vi "TapeMonitor_new.vi"() -> ()   [LabVIEW 2013]
uses:
  shared programs/GUI_Template/GUI_master/tcp_new_data_event.ctl
  shared programs/GUI_Template/GUI_master/tcp new data cluster.ctl
  <vilib>/vision/Image Controls.llb/IMAQ Image.ctl
  <vilib>/vision/NI_Vision_Development_Module.lvlib
  <vilib>/Analysis/NI_AALBase.lvlib
panel:
  out "x-y":dbl=0.8
  out "sqrt(x)":dbl=nan
  out "fitness":dbl=nan
  out "area symmetry":dbl=nan
  out "standard deviation":dbl=-0.0 format="%0.2f"
  out "Array":dbl[](array[numeric])
  out "symmetry":dbl=nan
  out "Number of Particles":i32
  out "X":dbl[](array[numeric])
  out "Y":dbl[](array[numeric])
  in  "Font, Size & Style":T1={"Desired Font (Application)"=enum."Application Font", "[User-specified Font]"={"Font Name"="", "Size"=12, "Strikeout?"=FALSE, "Italic?"=FALSE, "Underline?"=FALSE, "Outline?"=FALSE, "Shadow?"=FALSE, "Bold?"=FALSE, "Rotation Angle"=0.0}, "Horizontal Alignment"=0, "Vertical Alignment"=0} {"Vertical Alignment" items=["Bottom", "Top", "Baseline"]; "Horizontal Alignment" items=["Left", "Center", "Right"]; "[User-specified Font]"."Rotation Angle" format="%.2f"}
  in  "Selection Values":T3(array[cluster])=[{"Measurement Parameter"=35, "Range Lower Value"=0.0, "Range Upper Value"=500.0, "Range"=TRUE, "Measurement Type"=FALSE}] {"Measurement Parameter" items=["Center of Mass X", "Center of Mass Y", "First Pixel X", "First Pixel Y", "Bounding Rect Left", "Bounding Rect Top", "Bounding Rect Right", "Bounding Rect Bottom", "Max Feret Diameter Start X", "Max Feret Diameter Start Y", "Max Feret Diameter End X", "Max Feret Diameter End Y", "Max Horiz. Segment Length Left", "Max Horiz. Segment Length Right", "Max Horiz. Segment Length Row", "-", "Bounding Rect Width", "Bounding Rect Height", "Bounding Rect Diagonal", "Perimeter", "Convex Hull Perimeter", "Holes' Perimeter", "Max Feret Diameter", "Equivalent Ellipse Major Axis", "Equivalent Ellipse Minor Axis", "Equivalent Ellipse Minor Axis (Feret)", "Equivalent Rect Long Side", "Equivalent Rect Short Side", "Equivalent Rect Diagonal", "Equivalent Rect Short Side (Feret)", "Average Horiz. Segment Length", "Average Vert. Segment Length", "Hydraulic Radius", "Waddel Disk Diameter", "-", "Area", "Holes' Area", "Particle & Holes' Area", "Convex Hull Area", "Image Area", "-", "Number of Holes", "Number of Horiz. Segments", "Number of Vert. Segments", "-", "Orientation", "Max Feret Diameter Orientation", "-", "% Area/Image Area", "% Area/(Particle & Holes' Area)", "Ratio of Equivalent Ellipse Axes", "Ratio of Equivalent Rect Sides", "-", "Elongation Factor", "Compactness Factor", "Heywood Circularity Factor", "Type Factor", "-", "Sum X", "Sum Y", "Sum XX", "Sum XY", "Sum YY", "Sum XXX", "Sum XXY", "Sum XYY", "Sum YYY", "-", "Moment of Inertia XX", "Moment of Inertia XY", "Moment of Inertia YY", "Moment of Inertia XXX", "Moment of Inertia XXY", "Moment of Inertia XYY", "Moment of Inertia YYY", "Norm. Moment of Inertia XX", "Norm. Moment of Inertia XY", "Norm. Moment of Inertia YY", "Norm. Moment of Inertia XXX", "Norm. Moment of Inertia XXY", "Norm. Moment of Inertia XYY", "Norm. Moment of Inertia YYY", "Hu Moment 1", "Hu Moment 2", "Hu Moment 3", "Hu Moment 4", "Hu Moment 5", "Hu Moment 6", "Hu Moment 7"]}
  in  "Keep/Replace Value (Replace) 2":bool=TRUE
  out "image2":T4(plugin-control) caption="Mode1"
  in  "Size & Order # 2":T5={"X Size"=3, "Y Size"=3, "Order #"=8}
  in  "Range 2":cluster{"Lower value":sgl, "Upper value":sgl}={"Lower value"=140.0, "Upper value"=255.0} {"Upper value" format="%.2f"; "Lower value" format="%.2f"}
  in  "gain::1":dbl caption="gain" min=0.0 max=12.0 format="%_4p"
  out "image::1":T4(plugin-control) caption="Mode1"
  in  "exposure::1":dbl=0.01 caption="Exposure" min=0.0001 max=1.0 format="%_4p"
  in  "insert tag":bool=TRUE
  in  "stop":bool
  in  "trigger::1":bool caption="Trigger"
  in  "GUIdevice 1":string="StagingTapeMonitorCam"
  out "tcp data event":T6
  out "error IO 2":errorcluster
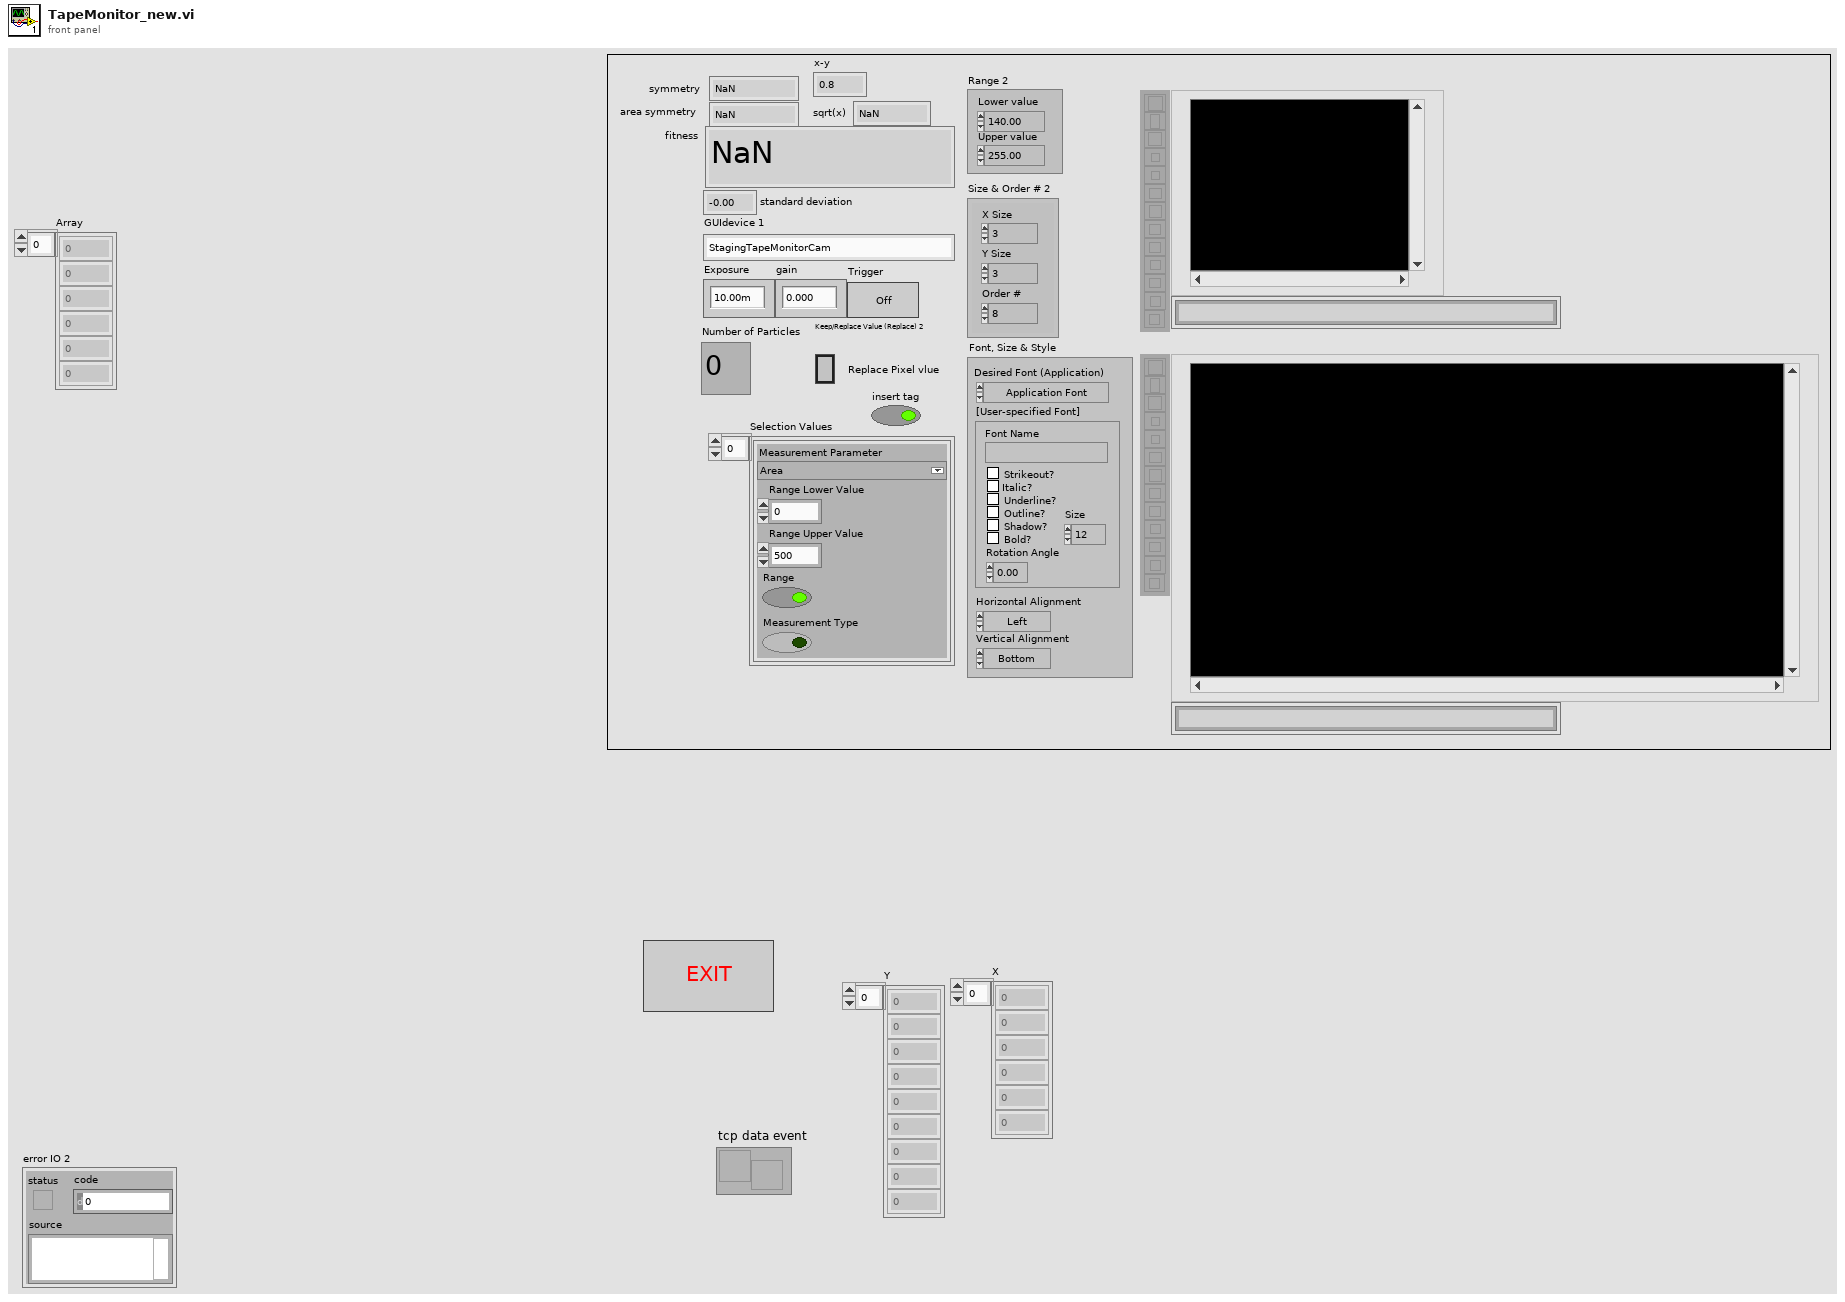
[diagram p1: front panel]
types:
  T1 = cluster{"Desired Font (Application)":enum16{"User-specified Font", "Application Font", "System Font", "Dialog Font"}, "[User-specified Font]":cluster{"Font Name":string, "Size":i16, "Strikeout?":bool, "Italic?":bool, "Underline?":bool, "Outline?":bool, "Shadow?":bool, "Bold?":bool, "Rotation Angle":dbl}, "Horizontal Alignment":i16, "Vertical Alignment":i16}
  T2 = typedef "Particle Parameters" = i32
  T3 = cluster{"Measurement Parameter":T2, "Range Lower Value":dbl, "Range Upper Value":dbl, "Range":bool, "Measurement Type":bool}[]
  T4 = typedef "IMAQ Image.ctl" = refnum<image>
  T5 = cluster{"X Size":i32, "Y Size":i32, "Order #":i32}
  T6 = typedef "tcp_new_data_event.ctl" = refnum<user-event>
  T7 = typedef "Image Type" = u32
  T8 = typedef "tcp new data cluster.ctl" = cluster{"EventEnum":enum16{"new data", "connection status update"}, "Device name":string}
  T9 = cluster{"Particle Measurements (Pixels)[0]":dbl, "Particle Measurements (Pixels)[1]":dbl, "Particle Measurements (Pixels)[2]":dbl, "Particle Measurements (Pixels)[3]":dbl}
  T10 = cluster{"Particle Measurements (Pixels)[0]":dbl, "Particle Measurements (Pixels)[1]":dbl}
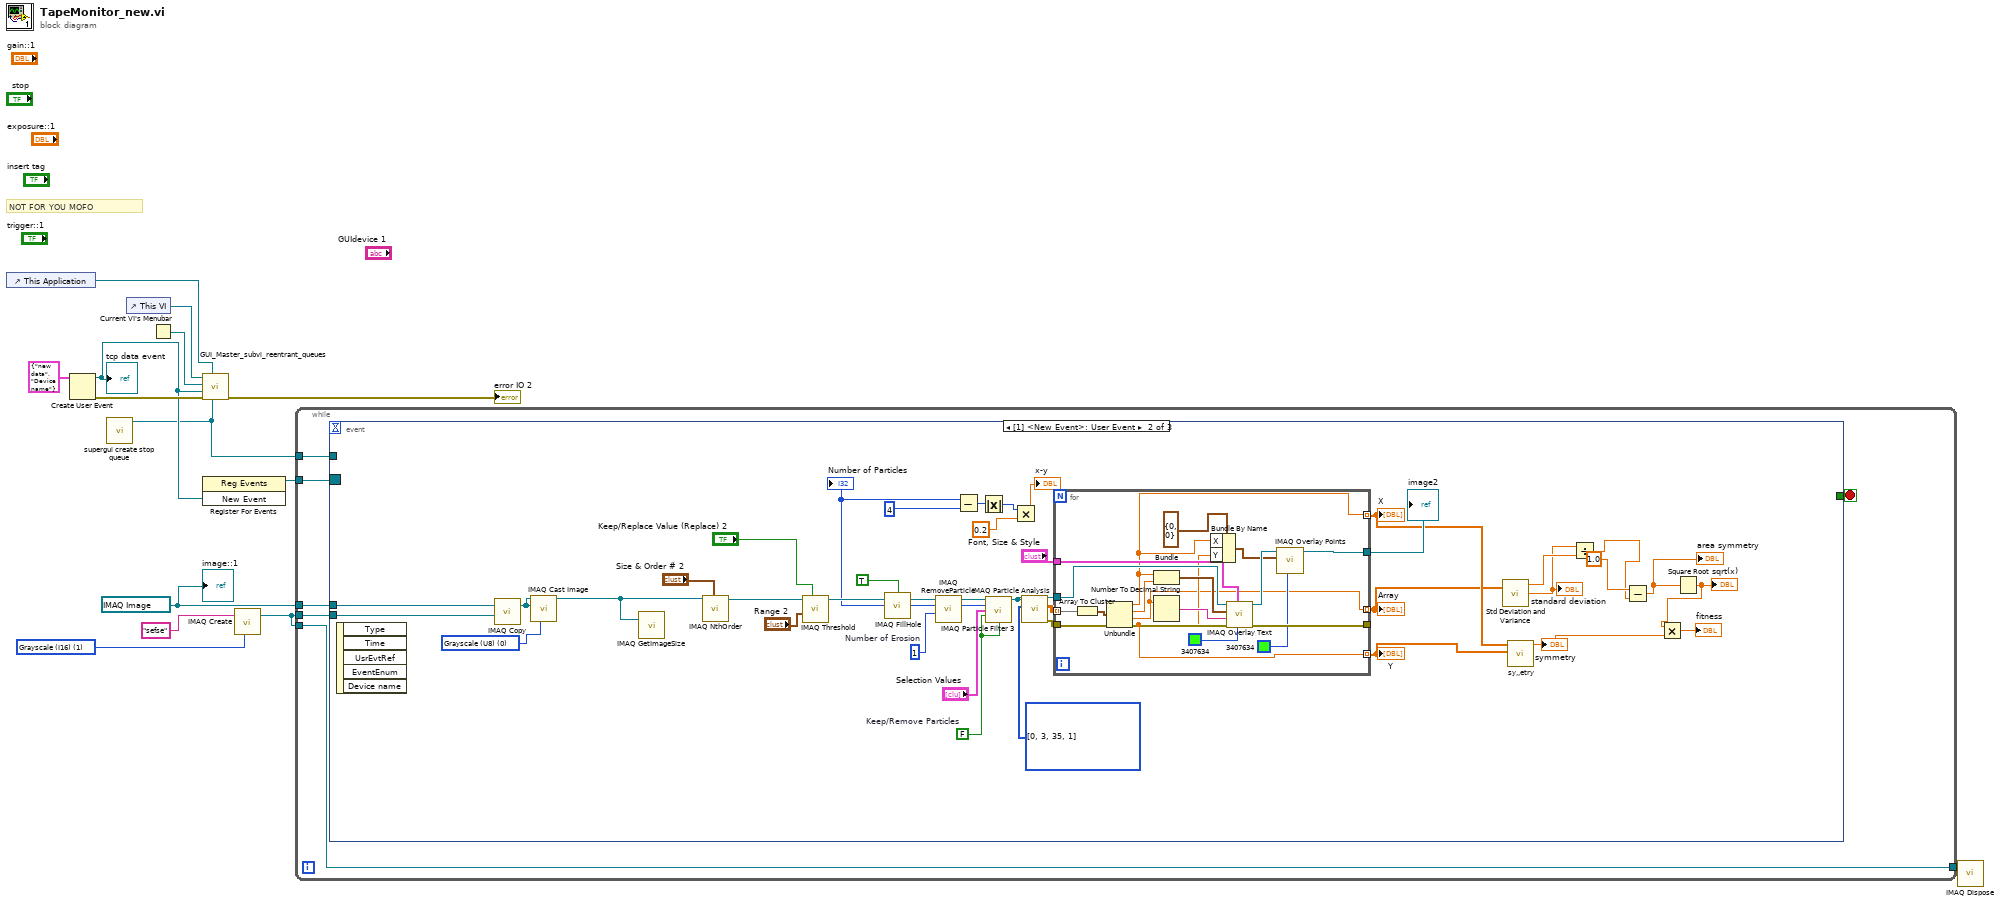
[diagram p0: block diagram]
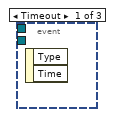
[diagram p2: hidden frame]
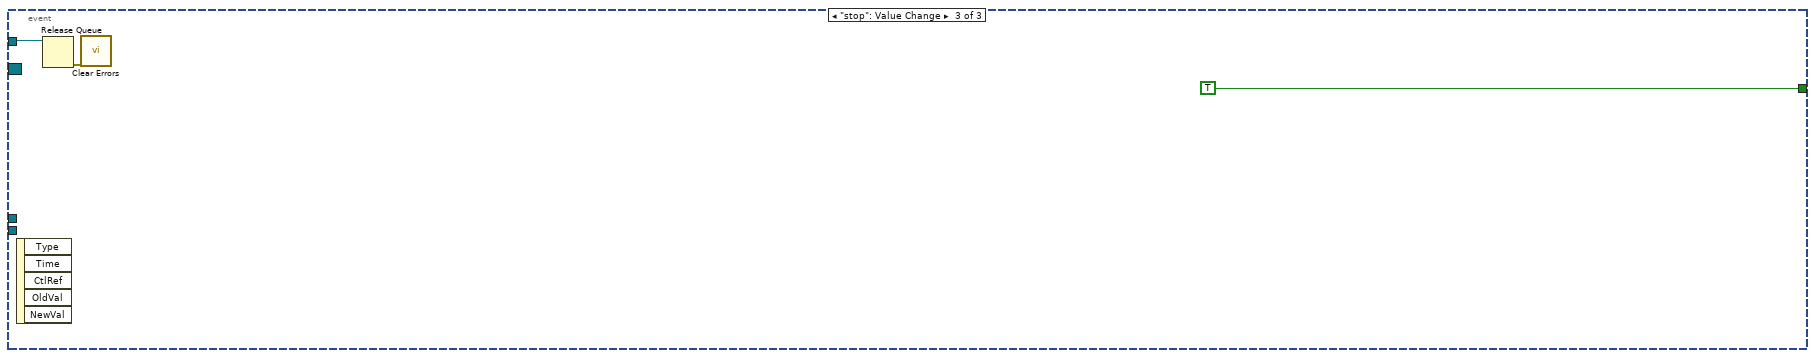
[diagram p3: hidden frame]
diagram:
  w6 = T7 1 items=["Grayscale (U8)", "Grayscale (I16)", "Grayscale (SGL)", "Complex (CSG)", "RGB (U32)", "HSL (U32)", "RGB (U64)", "Grayscale (U16)"] ("Image Type")
  w2 = T4 refnum ("New Image")
  # "NOT FOR YOU MOFO"
  n1 = control-ref of="This Application"() -> (w9:refnum<vi>)
  n2 = Create User Event(user event datatype=T8 {"EventEnum"=enum."new data", "Device name"="Device name"} ("New Event")) -> (user event=w7:refnum<user-event>, error out=w10:errorcluster)  [unwired: 1 in]
  "tcp data event" <- w7
  n3 = call "supergui create stop queue.vi"() -> ("STOP Queue out"=w1:refnum<queue>)  [unwired: 11 in]
  n4 = control-ref of="This VI"() -> (w13:refnum<vi>)
  n5 = Current VI's Menubar() -> (w12:refnum<k9>)
  n6 = call "GUI_Master_subvi_reentrant_queues.vi"("STOP Queue in"=w1, "This Application"=w9, "error in (no error)"=w10, "tcp data event"=w7, "Caller menu reference"=w12, "Caller VI ref"=w13) -> ("error out"=→"error IO 2":errorcluster)  [unwired: 5 in]
  n7 = register-events(w7) -> (reference out=w8:refnum<event-registration>)  [unwired: 2 in, 1 out]
  n8 = call "IMAQ Create"("Image Name"="sefse", "Image Type"=w6) -> ("New Image"=w4:T4)  [unwired: 3 in, 1 out]
  n9 = while {
    tunnel: w8 -> [w19]
    tunnel: w2 -> [w18]
    tunnel: w4 -> [w17]
    tunnel: w4 -> [w16]
    tunnel: [w16] -> w3
    tunnel: w1 -> [w15]
    stop <- w20 stop-if-true
    n10 = event shown="[1] <New Event>: User Event" {
      selector: w19 -> [_ _ _]
      dyn-events: _ -> [_ _ _]
      timeout: _ -> [_ _ _]
      tunnel: [_ _ TRUE] -> w20
      tunnel: w18 -> [_ w58 _]
      tunnel: w17 -> [_ w59 _]
      tunnel: w15 -> [_ _ w79]
      event Timeout {
        n11 = event-data() -> ()  [unwired: 1 in, 2 out]
      }
      event User Event {
        w39 = T2[] [0, 3, 35, 1] items=["Center of Mass X", "Center of Mass Y", "First Pixel X", "First Pixel Y", "Bounding Rect Left", "Bounding Rect Top", "Bounding Rect Right", "Bounding Rect Bottom", "Max Feret Diameter Start X", "Max Feret Diameter Start Y", "Max Feret Diameter End X", "Max Feret Diameter End Y", "Max Horiz. Segment Length Left", "Max Horiz. Segment Length Right", "Max Horiz. Segment Length Row", "-", "Bounding Rect Width", "Bounding Rect Height", "Bounding Rect Diagonal", "Perimeter", "Convex Hull Perimeter", "Holes' Perimeter", "Max Feret Diameter", "Equivalent Ellipse Major Axis", "Equivalent Ellipse Minor Axis", "Equivalent Ellipse Minor Axis (Feret)", "Equivalent Rect Long Side", "Equivalent Rect Short Side", "Equivalent Rect Diagonal", "Equivalent Rect Short Side (Feret)", "Average Horiz. Segment Length", "Average Vert. Segment Length", "Hydraulic Radius", "Waddel Disk Diameter", "-", "Area", "Holes' Area", "Particle & Holes' Area", "Convex Hull Area", "Image Area", "-", "Number of Holes", "Number of Horiz. Segments", "Number of Vert. Segments", "-", "Orientation", "Max Feret Diameter Orientation", "-", "% Area/Image Area", "% Area/(Particle & Holes' Area)", "Ratio of Equivalent Ellipse Axes", "Ratio of Equivalent Rect Sides", "-", "Elongation Factor", "Compactness Factor", "Heywood Circularity Factor", "Type Factor", "-", "Sum X", "Sum Y", "Sum XX", "Sum XY", "Sum YY", "Sum XXX", "Sum XXY", "Sum XYY", "Sum YYY", "-", "Moment of Inertia XX", "Moment of Inertia XY", "Moment of Inertia YY", "Moment of Inertia XXX", "Moment of Inertia XXY", "Moment of Inertia XYY", "Moment of Inertia YYY", "Norm. Moment of Inertia XX", "Norm. Moment of Inertia XY", "Norm. Moment of Inertia YY", "Norm. Moment of Inertia XXX", "Norm. Moment of Inertia XXY", "Norm. Moment of Inertia XYY", "Norm. Moment of Inertia YYY", "Hu Moment 1", "Hu Moment 2", "Hu Moment 3", "Hu Moment 4", "Hu Moment 5", "Hu Moment 6", "Hu Moment 7"] ("Pixel Measurements")
        w46 = FALSE  # Keep/Remove Particles
        w48 = 1  # Number of Erosion
        w55 = T7 0 items=["Grayscale (U8)", "Grayscale (I16)", "Grayscale (SGL)", "Complex (CSG)", "RGB (U32)", "HSL (U32)", "RGB (U64)", "Grayscale (U16)"] ("Image Type")
        n12 = event-data() -> ()  [unwired: 1 in, 5 out]
        n13 = call "IMAQ Copy"("Image Dst"=w59, "Image Src"=w58) -> ("Image Dst Out"=w57:T4)  [unwired: 4 in, 1 out]
        n14 = call "IMAQ Cast Image"("Image Type"=w55, "Image Dst"=w57, "Image Src"=w57) -> ("Image Dst Out"=w56:T4)  [unwired: 7 in, 1 out]
        n15 = call "IMAQ GetImageSize"("Image"=w56) -> ()  [unwired: 3 in, 3 out]
        n16 = call "IMAQ NthOrder"("Image Src"=w56, "Size & Order #"="Size & Order # 2") -> ("Image Dst Out"=w54:T4)  [unwired: 5 in, 1 out]
        n17 = call "IMAQ Threshold"("Keep/Replace Value (Replace)"="Keep/Replace Value (Replace) 2", "Range"="Range 2", "Image Src"=w54) -> ("Image Dst Out"=w50:T4)  [unwired: 7 in, 1 out]
        n18 = call "IMAQ FillHole"("Image Src"=w50, "Connectivity 4/8 (8)"=TRUE) -> ("Image Dst Out"=w49:T4)  [unwired: 2 in, 3 out]
        n19 = call "IMAQ RemoveParticle"("Number of Erosion"=w48, "Image Src"=w49) -> ("Image Dst Out"=w45:T4)  [unwired: 5 in, 4 out]
        n20 = call "IMAQ Particle Filter 3"("Image Src"=w45, "Selection Values"="Selection Values", "Keep/Remove Particles (F)"=w46, "Fill Holes? (F)"=w46) -> ("Image Dst Out"=w40:T4, "Number of Particles"=w26:i32)  [unwired: 5 in, 5 out]
        "Number of Particles" <- w26
        n21 = Subtract(x=w26, y=4) -> (x-y=w24:i32)
        n22 = Absolute Value(x=w24) -> (abs(x)=w23:i32)
        n23 = Multiply(x=w23, y=0.2) -> (x*y=→"x-y":dbl)
        n24 = call "IMAQ Particle Analysis"("Pixel Measurements"=w39, "Image"=w40) -> ("error out"=w41:errorcluster, "Particle Measurements (Pixels)"=w43:dbl[][])  [unwired: 3 in, 5 out]
        n25 = for {
          tunnel: w41 -> [w77]
          tunnel: [w76] -> _
          tunnel: [w66] -> w38
          tunnel: w40 -> [w73]
          tunnel: "Font, Size & Style" -> [w69]
          tunnel: w43 -> [w68] mode=indexing
          tunnel: [w62] -> w36 mode=indexing
          tunnel: [w61] -> w37 mode=indexing
          tunnel: [w60] -> w35 mode=indexing
          n26 = Array To Cluster(array=w68) -> (cluster=w72:T9)
          n27 = Unbundle(w72) -> ("Particle Measurements (Pixels)[0]"=w62:dbl, "Particle Measurements (Pixels)[1]"=w71:dbl, "Particle Measurements (Pixels)[2]"=w60:dbl, "Particle Measurements (Pixels)[3]"=w61:dbl)
          n28 = Bundle("Particle Measurements (Pixels)[0]"=w62, "Particle Measurements (Pixels)[1]"=w71) -> (w70:T10)  [unwired: 1 out]
          n29 = Number To Decimal String(number=w60) -> (decimal integer string=w75:string)  [unwired: 1 out]
          n30 = Bundle By Name(cluster=cluster{"X":i32, "Y":i32} {"X"=0, "Y"=0} ("Point"), "X"=w62, "Y"=w61) -> (w63:cluster{"X":i32, "Y":i32})
          n31 = call "IMAQ Overlay Text"("Text Color (black)"=u32 3407634, "Font, Size & Style"=w69, "error in (no error)"=w77, "String"=w75, "Origin"=w70, "Image"=w73) -> ("error out"=w76:errorcluster, "Image Out"=w67:T4)  [unwired: 2 in, 2 out]
          n32 = call "IMAQ Overlay Points"("Color"=u32 3407634 ("Text Color (black)"), "Point"=w63, "Image"=w67) -> ("Image Out"=w66:T4)  [unwired: 7 in, 1 out]
        }
        "image2" <- w38
        "Y" <- w37
        "X" <- w36
        "Array" <- w35
        n33 = call <vilib>:"Std Deviation and Variance.vi"("X"=w35) -> ("mean"=w34:dbl, "standard deviation"=w33:dbl)  [unwired: 1 in, 1 out]
        "standard deviation" <- w33
        n34 = call "sy,,etry.vi"("Array 2"=w37, "Array"=w36) -> ("x-y 3"=w30:dbl)  [unwired: 9 in]
        "symmetry" <- w30
        n35 = Divide(x=w33, y=w34) -> (x/y=w31:dbl)
        n36 = Subtract(x=1.0 ("x/y"), y=w31) -> (x-y=w28:dbl)
        "area symmetry" <- w28
        n37 = Square Root(x=w28) -> (sqrt(x)=w27:dbl)
        "sqrt(x)" <- w27
        n38 = Multiply(x=w27, y=w30) -> (x*y=→"fitness":dbl)
      }
      event "stop": Value Change {
        n39 = event-data() -> ()  [unwired: 1 in, 5 out]
        n40 = Release Queue(queue=w79) -> (error out=w78:errorcluster)  [unwired: 2 in, 2 out]
        n41 = call <vilib>:"Clear Errors.vi"("error in (no error)"=w78) -> ()  [unwired: 6 in, 1 out]
      }
    }
  }
  n42 = call "IMAQ Dispose"("Image"=w3) -> ()  [unwired: 5 in, 1 out]
  "image::1" <- w2
